vi "ConnectToHW(TriggeredMode).vi"(8 "error in (no error)":errorcluster, 11 "TektronixDPO in":refnum<class "TektronixDPO.lvclass">) -> (0 "error out":errorcluster, 3 "TektronixDPO out":refnum<class "TektronixDPO.lvclass">)   [LabVIEW 2013, in "TektronixDPO.lvclass"]
doc: "Connect to the scope and disable the continuous mode"
uses:
  TektronixDPO.lvclass
  SupportClasses/TektronixDPOPhysicalDevice/TektronixDPO_PhysicalDevice.lvclass
  TektronixDPO.lvclass/TektronixDPO.ctl
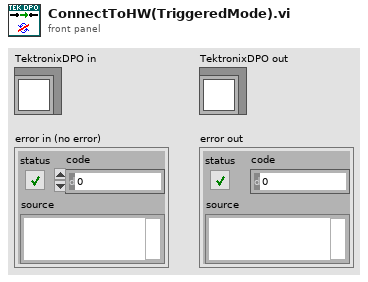
[diagram p1: front panel]
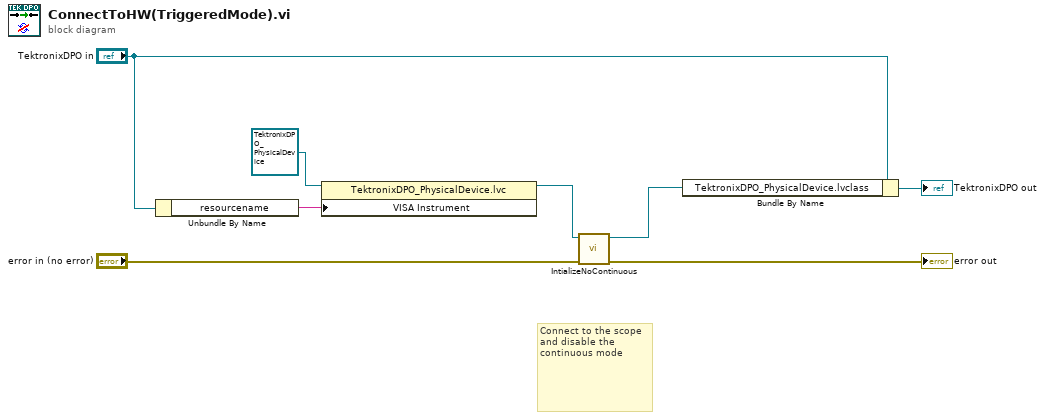
[diagram p0: block diagram]
diagram:
  # "Connect to the scope and disable the continuous mode"
  n1 = Unbundle By Name("TektronixDPO in") -> ("resourcename"=w3:string)
  n2 = property class="TektronixDPO_PhysicalDevice.lvc"(reference=refnum<class "TektronixDPO_PhysicalDevice.lvclass"> refnum ("TektronixDPO in"), "VISA Instrument"=w3) -> (reference out=w2:refnum<class "TektronixDPO_PhysicalDevice.lvclass">)  [unwired: 1 in, 1 out]
  n3 = call "IntializeNoContinuous.vi"("error in (no error)"="error in (no error)", "TektronixDPO_PhysicalDevice in"=w2) -> ("error out"=→"error out":errorcluster, "TektronixDPO_PhysicalDevice out"=w1:refnum<class "TektronixDPO_PhysicalDevice.lvclass">)  [unwired: 8 in]
  n4 = Bundle By Name(cluster="TektronixDPO in", "TektronixDPO_PhysicalDevice.lvclass"=w1) -> (→"TektronixDPO out":refnum<class "TektronixDPO.lvclass">)
